vi "PP_Demo.vi"(11 "String":string) -> ()   [LabVIEW 2014]
panel:
  out "error out":errorcluster {"code" format="%d\n0x%x"}
  in  "error in":errorcluster caption="error in (no error)" {"code" format="%d\n0x%x"}
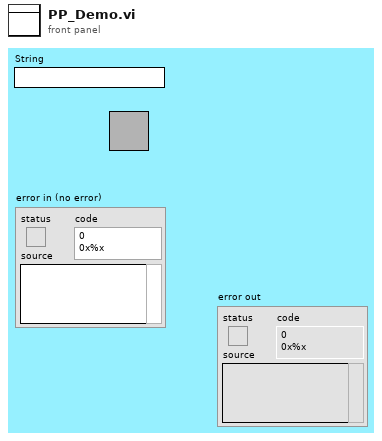
[diagram p1: front panel]
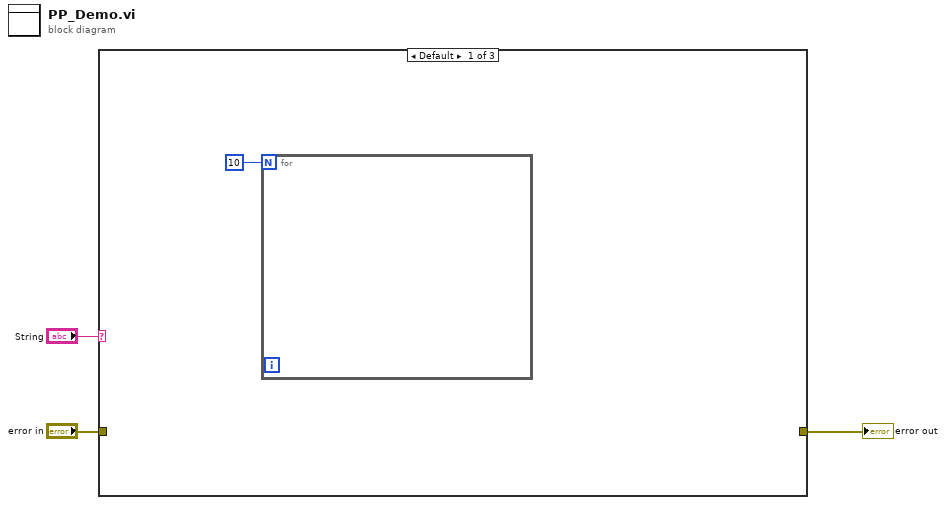
[diagram p0: block diagram]
diagram:
  n1 = case shown="Default" "String" {
    tunnel: [_ _ w5] -> w2
    tunnel: "error in" -> [_ _ w5]
    frame Default {
      n2 = for {
        N: 10 -> [_]
      }
    }
    frame "no Error" {
    }
    frame "Error" {
    }
  }
  "error out" <- w2
